vi "sample_a0.vi"(9 "threshold":i32, 11 "times":i32) -> (0 "布尔":bool, 3 "ai":sgl)   [LabVIEW 2012]
uses:
  <vilib>/eio/EIONode/EIONode.xnode
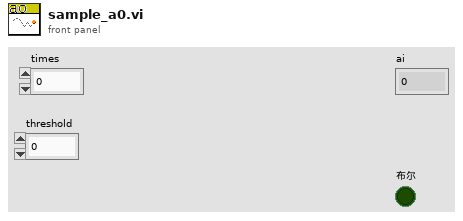
[diagram p1: front panel]
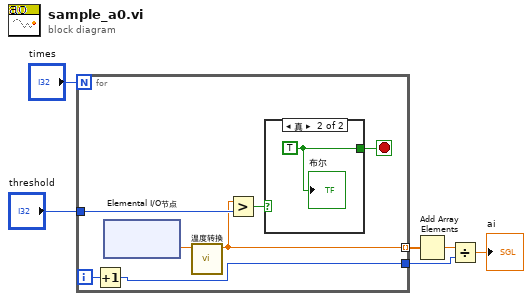
[diagram p0: block diagram]
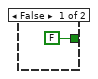
[diagram p2: hidden frame]
diagram:
  n1 = for {
    N: "times" -> [_]
    tunnel: [w9] -> w2 mode=indexing
    tunnel: "threshold" -> [w13]
    tunnel: [w7] -> w1
    i -> [w8]
    stop <- w11 stop-if-true
    n2 = Increment(x=w8) -> (x+1=w7:i32)
    n3 = xnode "Elemental I/O节点"() -> ("AI0"=w10:sgl)  [unwired: 1 in, 1 out]
    n4 = call "温度转换.vi"("in"=w10) -> ("out"=w9:dbl)  [unwired: 10 in]
    n5 = Greater?(x=w9, y=w13) -> (0:w12:bool)
    n6 = case shown="真" w12 {
      tunnel: [FALSE ("布尔") w15] -> w11
      frame False {
      }
      frame True {
        w15 = TRUE ("布尔")
        "布尔" <- w15
      }
    }
  }
  n7 = Add Array Elements(numeric array=w2) -> (sum=w6:dbl)
  n8 = Divide(x=w6, y=w1) -> (x/y=→"ai":dbl)
